vi "WorkerFactory.vi"(8 "error in (no error)":errorcluster, 11 "BuildWorker in":refnum<class "BuildWorker.lvclass">) -> (0 "error out":errorcluster, 1 "Port":u16, 2 "BuildWorkers":refnum<class "BuildWorker.lvclass">[](array[class]), 3 "BuildWorker out":refnum<class "BuildWorker.lvclass">, 4 "Show":bool)   [LabVIEW 2017, in "BuildWorker Interface.lvlib" / "BuildWorker.lvclass"]
uses:
  BuildWorker.lvclass
  BuildWorker.lvclass/BuildWorker.ctl
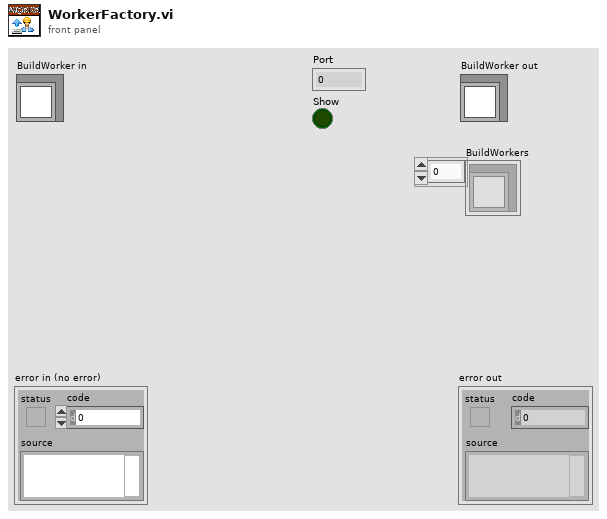
[diagram p1: front panel]
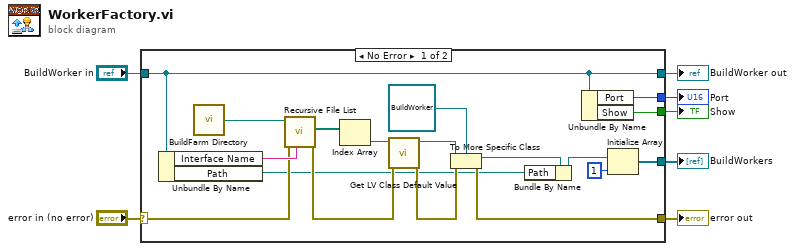
[diagram p0: block diagram]
diagram:
  n1 = case shown="No Error" "error in (no error)" {
    selector: "error in (no error)" -> [w24 w27]
    tunnel: [w18 w27] -> w6
    tunnel: [w15 w26] -> w4
    tunnel: "BuildWorker in" -> [w15 w26]
    tunnel: [w16 _] -> w3
    tunnel: [w13 _] -> w2
    tunnel: [w12 _] -> w1
    frame No Error {
      n2 = Unbundle By Name(w15) -> ("Interface Name"=w25:string, "Path"=w9:path)
      n3 = call "BuildFarm Directory.vi"() -> ("BuildFarm Directory"=w8:path)
      n4 = call <vilib>:"Recursive File List.vi"("pattern"=w25, "error in (no error)"=w24, "Folder Path"=w8) -> ("error out"=w21:errorcluster, "All Files in Dir"=w23:path[])  [unwired: 4 in, 3 out]
      n5 = Index Array(array=w23) -> (element=w22:path)  [unwired: 1 in]
      n6 = call <vilib>:"Get LV Class Default Value.vi"("error in (no error)"=w21, "class path"=w22) -> ("error out"=w20:errorcluster, "object"=w19:refnum<class>)  [unwired: 8 in]
      n7 = To More Specific Class(target class=refnum<class "BuildWorker.lvclass"> refnum ("BuildWorker Controller.lvlib:BuildWorker.lvclass"), reference=w19, error in=w20) -> (specific class reference=w14:refnum<class "BuildWorker.lvclass">, error out=w18:errorcluster)
      n8 = Bundle By Name(cluster=w14, "Path"=w9) -> (w10:refnum<class "BuildWorker.lvclass">)
      n9 = Unbundle By Name(w15) -> ("Port"=w13:u16, "Show"=w12:bool)
      n10 = Initialize Array(w10, 1 ("dimension size")) -> (w16:refnum<class "BuildWorker.lvclass">[])
    }
    frame Error {
    }
  }
  "error out" <- w6
  "BuildWorker out" <- w4
  "BuildWorkers" <- w3
  "Port" <- w2
  "Show" <- w1
